vi "Walk measure_AFM.vi"() -> ()   [LabVIEW 2021]
uses:
  <userlib>/Nanonis Prog Interface V5/Nanonis Prog Interface.lvlib
panel:
  out "Delta reached?":bool
  out "Cap reached?":bool
  in  "Cap threshold (pA)":dbl
  in  "Delta cap threshold (pA)":dbl
  in  "pause":bool
  in  "Delete First Entry":bool
  in  "Time between averages (ms)":u32
  out "Avg index":i32
  in  "Averages":i32=50
  in  "milliseconds to wait":u32=1000
  in  "stop":bool
  in  "?":bool
  in  "Max Steps":u16=500
  in  "Direction":enum16{"X +", "X -", "Y +", "Y -", "Z +", "Z -"}(ring)
  out "Delta":cluster{"index":i32, sgl}[](graph)
  in  "Number of Steps":u16=50
  out "Capacitance":cluster{"index":i32, sgl}[](graph)
  in  "Frequency (Hz)":sgl=261.0
  in  "Amplitude (V)":sgl=260.0
  # "KPN: CORRECT NAVIGATION PROGRAM, 6/12/22"
  # "Threshold only works \nin Z+ direction"
  # "Max Steps On"
  # "Max Steps Off"
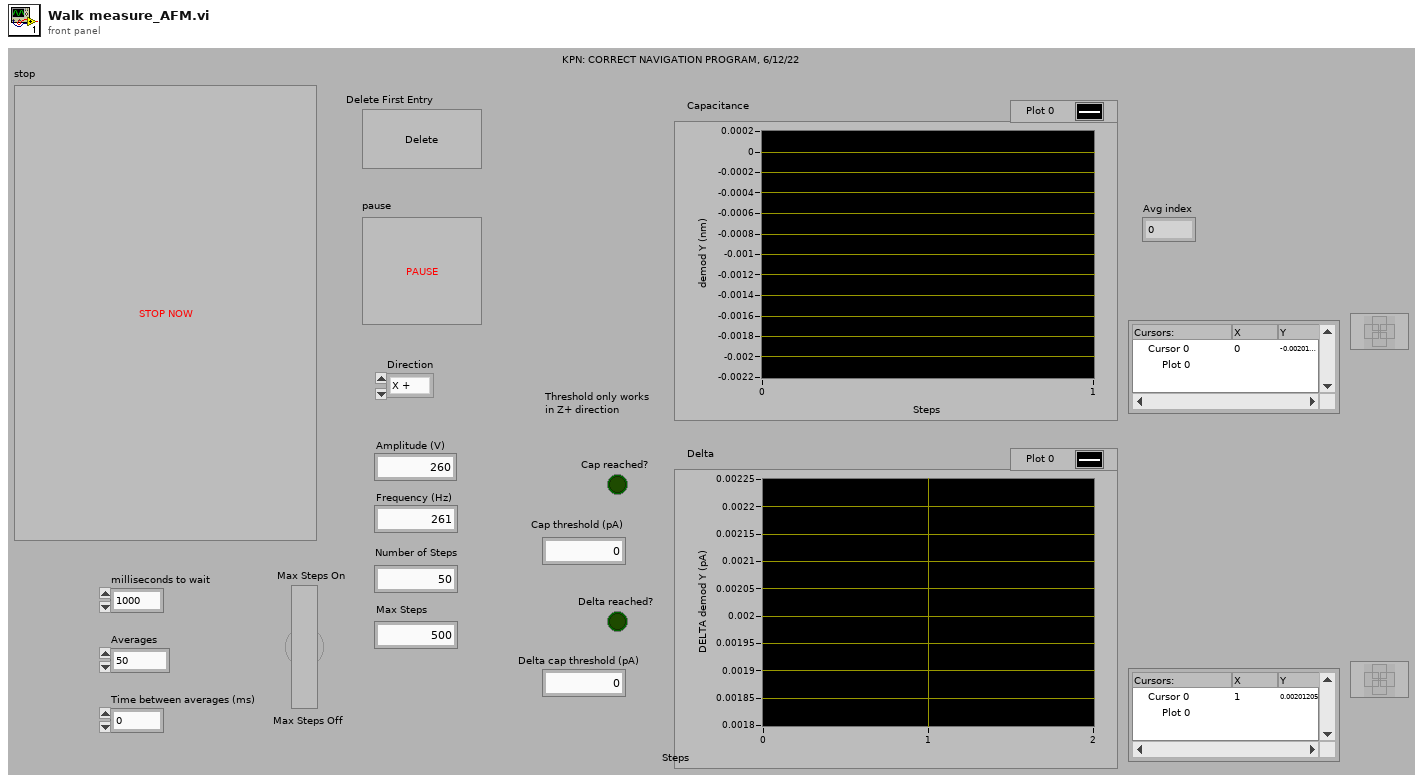
[diagram p1: front panel]
types:
  T1 = enum8{"Group 1", "Group 2", "Group 3", "Group 4", "Group 5", "Group 6"}
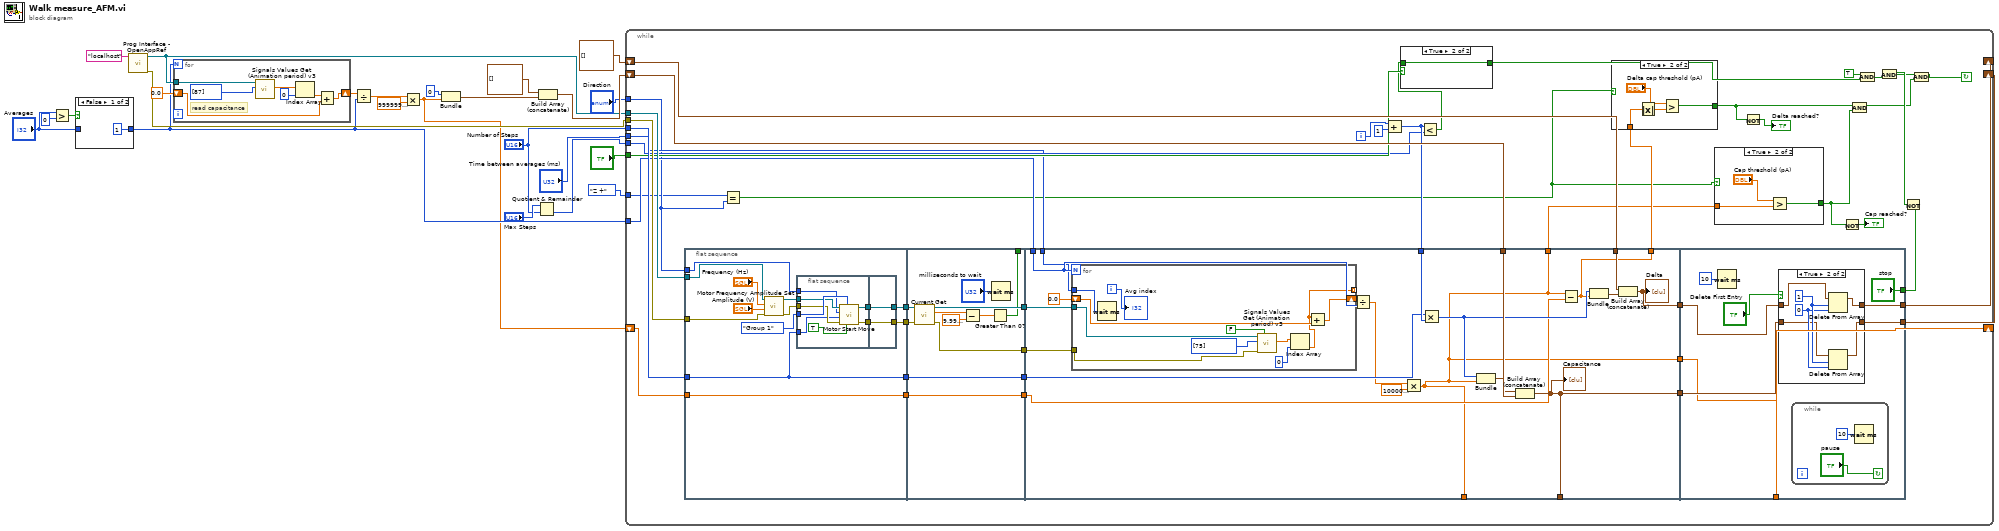
[diagram p0: block diagram]
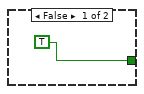
[diagram p3: hidden frame]
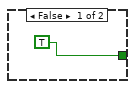
[diagram p4: hidden frame]
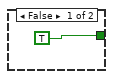
[diagram p5: hidden frame]
diagram:
  n1 = Greater?(x="Averages", y=0) -> (0:w9:bool)
  n2 = case shown="False" w9 {
    tunnel: "Averages" -> [_ w26]
    tunnel: [1 ("Averages") w26] -> w4
    frame False {
    }
    frame True {
    }
  }
  n3 = call <userlib>:"Prog Interface - OpenAppRef.vi"("Machine name (local machine IP)"="localhost" ("machine name (localhost)")) -> ("Error out"=w18:errorcluster, "Application reference"=w17:refnum<vi>)  [unwired: 5 in]
  n4 = for {
    N: w4 -> [_]
    tunnel: w17 -> [w30]
    shift-right: [w27] -> w5
    shift-left: sgl 0.0 ("Internal Ch Value") -> [w29]
    # "read capacitance"
    n5 = call <userlib>:"Signals Values Get (Animation period) v3.vi"("Signals indexes (0-127)"=i8[] [87], "Application ref in"=w30) -> ("Signals Values"=w31:sgl[])  [unwired: 6 in, 2 out]
    n6 = Index Array(array=w31, index=0) -> (element=w28:sgl)
    n7 = Add(x=w28, y=w29) -> (x+y=w27:sgl)
  }
  n8 = Divide(x=w5, y=w4) -> (x/y=w3:sgl)
  n9 = Multiply(x=w3, y=sgl 1000000000000.0) -> (x*y=w2:sgl)
  n10 = Bundle("index"=0, w2) -> (w21:cluster{"index":i32, sgl})  [unwired: 1 in]
  n11 = Quotient & Remainder(x="Max Steps", y="Number of Steps") -> (floor(x/y)=w12:u16)  [unwired: 1 out]
  n12 = Build Array (concatenate)(cluster{i32, sgl}[] [], w21) -> (w20:cluster{"index":i32, sgl}[])
  n13 = while {
    shift-right: [w50] -> _
    shift-left: w20 -> [w76]
    tunnel: w17 -> [w74]
    tunnel: w18 -> [w73]
    shift-right: [w67] -> _
    shift-left: cluster{i32, sgl}[] [] -> [w66]
    tunnel: "Direction" -> [w36]
    tunnel: "Number of Steps" -> [w65]
    tunnel: w12 -> [w58]
    tunnel: "?" -> [w64]
    tunnel: w4 -> [w53]
    tunnel: "Time between averages (ms)" -> [w52]
    shift-right: [w48] -> _
    shift-left: w2 -> [w47]
    tunnel: enum16{"X +", "X -", "Y +", "Y -", "Z +", "Z -"}."Z +" ("Direction") -> [w35]
    i -> [w61]
    stop <- w43 continue-if-true
    n14 = flat-sequence {
      tunnel: [w92] -> w78
      tunnel: w74 -> [w95]
      tunnel: w73 -> [w98]
      tunnel: [w97] -> w72
      tunnel: [w96] -> w71
      tunnel: w36 -> [w91]
      tunnel: w65 -> [w92]
      tunnel: w47 -> [w90]
      tunnel: [w90] -> w46
      tunnel: w78 -> [w124]
      tunnel: [w124] -> w77
      tunnel: w72 -> [w123]
      tunnel: w71 -> [w122]
      tunnel: [w121] -> w70
      tunnel: [w120] -> w69
      tunnel: [w117] -> _
      tunnel: w46 -> [w114]
      tunnel: [w114] -> w45
      tunnel: [w128] -> _
      tunnel: w59 -> [w143]
      tunnel: w77 -> [w140]
      tunnel: w76 -> [w141]
      tunnel: [w125] -> _
      tunnel: w70 -> [w139]
      tunnel: w69 -> [w138]
      tunnel: [w134] -> w68
      tunnel: w66 -> [w135]
      tunnel: w53 -> [w130]
      tunnel: w52 -> [w129]
      tunnel: [w128] -> w51
      tunnel: [w125] -> w49
      tunnel: w45 -> [w127]
      tunnel: [w126] -> w44
      tunnel: [w125] -> w42
      tunnel: w68 -> [w161]
      tunnel: [w160] -> w67
      tunnel: ["stop"] -> w54
      tunnel: [w158] -> w50
      tunnel: w51 -> [w159]
      tunnel: w49 -> [w157]
      tunnel: [w157] -> w48
      frame #0 {
        n15 = call <userlib>:"Motor Frequency Amplitude Set.vi"("Error in (no error)"=w98, "Amplitude (V) (NaN=no change)"="Amplitude (V)", "Frequency (Hz) (NaN=no change)"="Frequency (Hz)", "Application ref in"=w95) -> ("Error out"=w99:errorcluster, "Application ref out"=w100:refnum<vi>)  [unwired: 6 in]
        n16 = flat-sequence {
          tunnel: T1."Group 1" ("Group") -> [w110]
          tunnel: w100 -> [w109]
          tunnel: w99 -> [w108]
          tunnel: w92 -> [w107]
          tunnel: [w106] -> w94
          tunnel: [w105] -> w93
          tunnel: w91 -> [w104]
          tunnel: [w112] -> w96
          tunnel: [w113] -> w97
          tunnel: w94 -> [w113]
          tunnel: w93 -> [w112]
          frame #0 {
            n17 = call <userlib>:"Motor Start Move.vi"("Wait until finished? (F)"=TRUE, "Group"=w110, "Error in (no error)"=w108, "Number of steps"=w107, "Direction"=w104, "Application ref in"=w109) -> ("Error out"=w105:errorcluster, "Application ref out"=w106:refnum<vi>)  [unwired: 3 in]
          }
          frame #1 {
          }
        }
      }
      frame #1 {
        n18 = call <userlib>:"Current Get.vi"("Error in (no error)"=w122, "Application ref in"=w123) -> ("Error out"=w121:errorcluster, "Current (A)"=w119:sgl, "Application ref out"=w120:refnum<vi>)  [unwired: 5 in]
        n19 = Subtract(x=w119, y=sgl 1e-09) -> (x-y=w118:sgl)
        n20 = Greater Than 0?(x=w118) -> (x > 0?=w117:bool)
        n21 = Wait (ms)(milliseconds to wait="milliseconds to wait") -> ()  [unwired: 1 out]
      }
      frame #2 {
        n22 = for {
          N: w130 -> [_]
          tunnel: w139 -> [w148]
          tunnel: w138 -> [w147]
          shift-right: [w154] -> w132
          shift-left: sgl 0.0 ("y") -> [w155]
          tunnel: w129 -> [w152]
          tunnel: [w149] -> _ mode=indexing
          i -> [w153]
          n23 = Wait (ms)(milliseconds to wait=w152) -> ()  [unwired: 1 out]
          n24 = call <userlib>:"Signals Values Get (Animation period) v3.vi"("Wait for newest data (F=False)"=FALSE, "error in (no error)"=w148, "Signals indexes (0-127)"=i8[] [75], "Application ref in"=w147) -> ("Signals Values"=w151:sgl[])  [unwired: 4 in, 2 out]
          n25 = Index Array(array=w151, index=0) -> (element=w149:sgl)
          n26 = Add(x=w149, y=w155) -> (x+y=w154:sgl)
          "Avg index" <- w153
        }
        n27 = Divide(x=w132, y=w130) -> (x/y=w131:sgl)
        n28 = Multiply(x=w131, y=sgl 1000000000.0) -> (x*y=w125:sgl)
        n29 = Multiply(x=w140, y=w143) -> (x*y=w137:i32)
        n30 = Bundle(w137, w125) -> (w142:cluster{i32, sgl})  [unwired: 1 in]
        n31 = Build Array (concatenate)(w141, w142) -> (w128:cluster{"index":i32, sgl}[])
        "Capacitance" <- w128
        n32 = Subtract(x=w125, y=w127) -> (x-y=w126:sgl)
        n33 = Bundle(w137, w126) -> (w136:cluster{i32, sgl})  [unwired: 1 in]
        n34 = Build Array (concatenate)(w135, w136) -> (w134:cluster{i32, sgl}[])
        "Delta" <- w134
      }
      frame #3 {
        n35 = Wait (ms)(milliseconds to wait=u32 10) -> ()  [unwired: 1 out]
        n36 = case shown="True" "Delete First Entry" {
          tunnel: w161 -> [w167 w171]
          tunnel: [w167 w170] -> w160
          tunnel: w159 -> [w166 w168]
          tunnel: [w166 w169] -> w158
          frame False {
          }
          frame True {
            w173 = 1 ("length")
            w172 = 0 ("index")
            n37 = Delete From Array(array=w171, length=w173, index=w172) -> (array with subset deleted=w170:cluster{i32, sgl}[])  [unwired: 1 out]
            n38 = Delete From Array(array=w168, length=w173, index=w172) -> (array with subset deleted=w169:cluster{"index":i32, sgl}[])  [unwired: 1 out]
          }
        }
        n39 = while {
          stop <- "pause" continue-if-true
          n40 = Wait (ms)(milliseconds to wait=u32 10) -> ()  [unwired: 1 out]
        }
      }
    }
    n41 = Equal?(x=w35, y=w36) -> (x = y?=w34:bool)
    n42 = Add(x=w61, y=u16 1) -> (x+y=w59:i32)
    n43 = Less?(x=w59, y=w58) -> (x < y?=w60:bool)
    n44 = case shown="True" w64 {
      tunnel: w60 -> [_ w89]
      tunnel: [TRUE w89] -> w62
      frame False {
      }
      frame True {
      }
    }
    n45 = case shown="True" w34 {
      tunnel: w44 -> [_ w87]
      tunnel: [TRUE w85] -> w40
      frame False {
      }
      frame True {
        n46 = Absolute Value(x=w87) -> (abs(x)=w84:sgl)
        n47 = Greater?(x="Delta cap threshold (pA)", y=w84) -> (0:w85:bool)
      }
    }
    n48 = case shown="True" w34 {
      tunnel: w42 -> [_ w81]
      tunnel: [TRUE w80] -> w38
      frame False {
      }
      frame True {
        n49 = Greater?(x="Cap threshold (pA)", y=w81) -> (0:w80:bool)
      }
    }
    n50 = Not(x=w40) -> (.not. x?=→"Delta reached?":bool)
    n51 = Not(x=w38) -> (.not. x?=→"Cap reached?":bool)
    n52 = And(x=w40, y=w38) -> (x .and. y?=w41:bool)
    n53 = And(x=TRUE, y=w62) -> (x .and. y?=w56:bool)
    n54 = Not(x=w54) -> (.not. x?=w57:bool)
    n55 = And(x=w57, y=w56) -> (x .and. y?=w55:bool)
    n56 = And(x=w55, y=w41) -> (x .and. y?=w43:bool)
  }
